vi "ATF Storage-AI_Scale_Config.vi"(8 "error in (no error)":errorcluster, 10 "AI C":T1(array[cluster]), 11 "Refnum in":refnum<k21>) -> (0 "error out":errorcluster, 3 "Refnum out":refnum<k21>)   [LabVIEW 2022 SP3]
uses:
  <vilib>/DAQmx/create/scale.llb/DAQmx Create Scale (Map Ranges).vi
  <vilib>/DAQmx/create/channels.llb/DAQmx Create Channel (AI-Current-Basic).vi
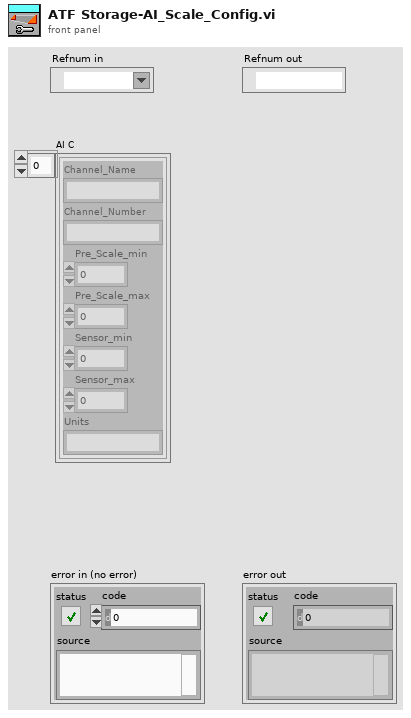
[diagram p1: front panel]
types:
  T1 = cluster{"Channel_Name":string, "Channel_Number":string, "Pre_Scale_min":dbl, "Pre_Scale_max":dbl, "Sensor_min":dbl, "Sensor_max":dbl, "Units":string}[]
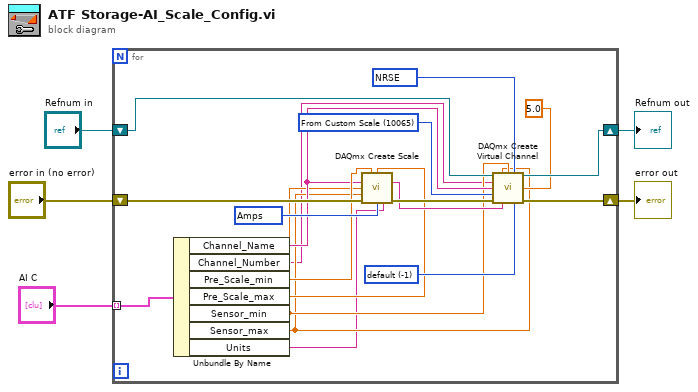
[diagram p0: block diagram]
diagram:
  n1 = for {
    shift-right: [w23] -> w3
    shift-left: "Refnum in" -> [w24]
    shift-right: [w21] -> w2
    shift-left: "error in (no error)" -> [w16]
    tunnel: "AI C" -> [w6] mode=indexing
    w14 = -1 items=["default"=-1, "Internal"=10200, "External"=10167] ("shunt resistor location")
    w17 = 10065 items=["Volts"=10348, "From Custom Scale"=10065] ("units")
    w18 = 10078 items=["Default"=-1, "RSE"=10083, "NRSE"=10078, "Differential"=10106, "Pseudodifferential"=12529] ("input terminal configuration")
    w20 = 10342 items=["Volts"=10348, "Amps"=10342, "Deg F"=10144, "Deg C"=10143, "Deg R"=10145, "Kelvins"=10325, "Strain"=10299, "Ohms"=10384, "Hz"=10373, "Seconds"=10364, "Meters"=10219, "Inches"=10379, "Degrees"=10146, "Radians"=10273, "Ticks"=10304, "g"=10186, "m/s^2"=12470, "m/s"=15959, "in/s"=15960, "Pascals"=10081, "Newtons"=15875, "Pounds"=15876, "kgf"=15877, "psi"=15879, "bar"=15880, "Nm"=15881, "oz-in"=15882, "lb-in"=15883, "lb-ft"=15884, "Volts/Volt"=15896, "mVolts/Volt"=15897, "pCoulombs"=16103, "Coulombs"=16102, "From TEDS"=12516] ("pre-scaled units")
    n2 = Unbundle By Name(w6) -> ("Channel_Name"=w11:string, "Channel_Number"=w8:string, "Pre_Scale_min"=w13:dbl, "Pre_Scale_max"=w12:dbl, "Sensor_min"=w10:dbl, "Sensor_max"=w9:dbl, "Units"=w7:string)
    n3 = call-poly <vilib>:"DAQmx Create Scale.vi"("pre-scaled minimum"=w13, "pre-scaled maximum"=w12, "name"=w11, "scaled minimum"=w10, "scaled maximum"=w9, "error in"=w16, "pre-scaled units"=w20, "scaled units"=w7) -> ("scale out"=w19:tag, "error out"=w22:errorcluster)  [unwired: 6 in]
    n4 = call-poly <vilib>:"DAQmx Create Virtual Channel.vi"("task in"=w24, "maximum value"=w9, "minimum value"=w10, "input terminal configuration"=w18, "physical channels"=w8, "name to assign"=w11, "external shunt resistor value"=5.0, "units"=w17, "error in"=w22, "custom scale name"=w19, "shunt resistor location"=w14) -> ("task out"=w23:refnum<k21>, "error out"=w21:errorcluster)  [unwired: 3 in]
  }
  "Refnum out" <- w3
  "error out" <- w2
